vi "Detect AprilTags.vi"() -> ()   [LabVIEW 2020, in "examples.lvlib"]
doc: "Demonstrate the AprilTag Detector and the utilities for getting AprilTag Family Image Data."
uses:
  examples.lvlib
  feature_detection/Apriltag Detector/AprilTag Detector.lvclass/AprilTag Detector.ctl
  feature_detection/Apriltag Detector/AprilTag Detector.lvclass
  image/image.lvlib
  image/ARGB Colour.ctl
  feature_detection/feature_detection.lvlib
  image/Draw Poly Lines (ARGB).vi
  image/Draw Image to Picture (ARGB).vi
  image/New Image (ARGB Preallocated).vi
  feature_detection/Apriltag Detector/Create (Tag36h11).vi
  image/Horizontal Concat Image Data (ARGB).vi
  feature_detection/AprilTag ID List (Tag36h11).vi
  feature_detection/Generate Apriltag Image Data (Tag36h11).vi
  image/New Image (Greyscale Array).vi
  common/Image Point (Float).ctl
  common/common.lvlib
  common/Quad Corners.ctl
  feature_detection/Apriltag Detector/Detection.ctl
  feature_detection/Apriltag Detector/Time Profiler Entry.ctl
panel:
  out "Time Profile Entries":T1[](array[typedef])
  out "Picture":picture
  out "Detections":T2[](array[typedef])
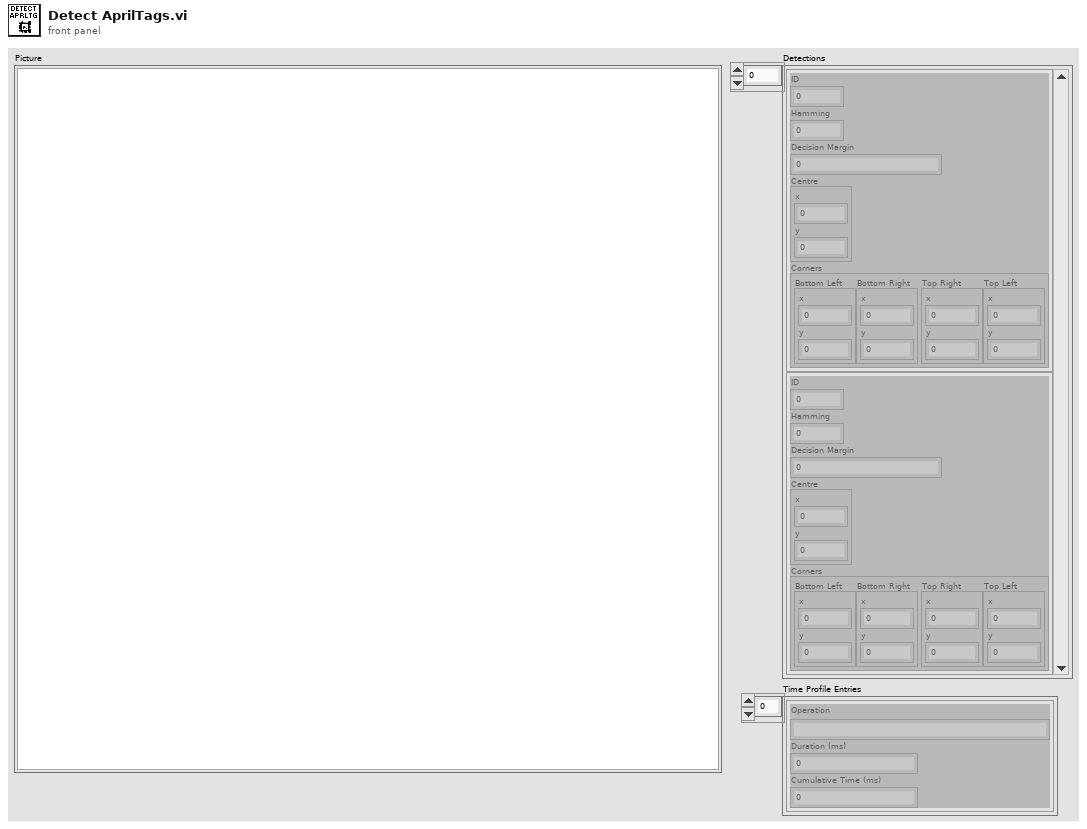
[diagram p1: front panel]
types:
  T1 = typedef "feature_detection.lvlib/AprilTag Detector.lvclass/Time Profiler Entry.ctl" = cluster{"Operation":string, "Duration (ms)":dbl, "Cumulative Time (ms)":dbl}
  T2 = typedef "feature_detection.lvlib/AprilTag Detector.lvclass/Detection.ctl" = cluster{"ID":i32, "Hamming":i32, "Decision Margin":sgl, "Centre":T3, "Corners":T4}
  T3 = typedef "common.lvlib/Image Point (Float).ctl" = cluster{"x":dbl, "y":dbl}
  T4 = typedef "common.lvlib/Quad Corners.ctl" = cluster{"Bottom Left":T3, "Bottom Right":T3, "Top Right":T3, "Top Left":T3}
  T5 = typedef "image.lvlib/ARGB Colour.ctl" = cluster{"Alpha":u8, "RGB":u32}
  T6 = typedef "image.lvlib/Greyscale Image.ctl" = refnum<data-value>
  T7 = typedef "image.lvlib/ARGB Image.ctl" = refnum<data-value>
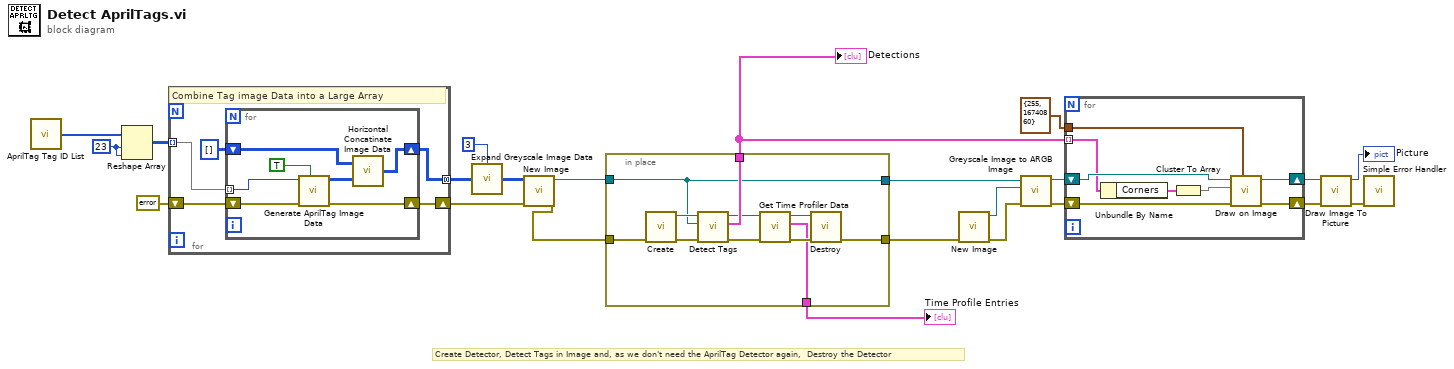
[diagram p0: block diagram]
diagram:
  w8 = 23 ("dimension size")
  # "Create Detector, Detect Tags in Image and, as we don't need the AprilTag Detector again,  Destroy the Detector"
  n1 = call-poly "AprilTag Tag ID List.vi"() -> ("Tag IDs"=w10:i32[])
  n2 = Reshape Array(w10, w8, w8) -> (w9:i32[][])
  n3 = for {
    tunnel: w9 -> [w28] mode=indexing
    tunnel: [w24] -> w6 mode=concatenating
    shift-right: [w26] -> w7
    shift-left: errorcluster {"status"=FALSE, "code"=0, "source"=""} ("error out") -> [w27]
    # "Combine Tag image Data into a Large Array"
    n4 = for {
      tunnel: w28 -> [w35] mode=indexing
      shift-right: [w33] -> w26
      shift-left: w27 -> [w34]
      shift-right: [w29] -> w24
      shift-left: u8[][] [] ("A") -> [w30]
      n5 = call-poly "Generate AprilTag Image Data.vi"("Add Border (Default: False)"=TRUE, "error in (no error)"=w34, "ID"=w35) -> ("error out"=w33:errorcluster, "Tag Image Data"=w31:u8[][])  [unwired: 7 in]
      n6 = call-poly "Horizontal Concatinate Image Data.vi"("B"=w31, "A"=w30) -> ("A Horizontal Concatinated with B"=w29:u8[][])
    }
  }
  n7 = call "Expand Greyscale Image Data.vi"("Greyscale Data"=w6, "Factor"=u16 3) -> ("Expanded Greyscale Data"=w5:u8[][])
  n8 = call-poly "New Image.vi"("error in (no error)"=w7, "U8 Greyscale Data"=w5) -> ("error out"=w23:errorcluster, "Greyscale Image"=w22:T6)  [unwired: 8 in]
  n9 = in-place {
    in-place-border: w23 -> [w45]
    in-place-border: w22 -> [w41]
    in-place-border: [w44] -> w21
    in-place-border: [w43] -> w16
    in-place-border: [w41] -> w2
    in-place-border: [w36] -> w1
    n10 = call-poly "Create.vi"("error in (no error)"=w45) -> ("error out"=w42:errorcluster, "Apriltag Detector"=w46:refnum<class "AprilTag Detector.lvclass">)  [unwired: 9 in]
    n11 = call "Detect Tags.vi"("error in (no error)"=w42, "Greyscale Image in"=w41, "Apriltag Detector in"=w46) -> ("error out"=w39:errorcluster, "Detections"=w43:T2[], "Apriltag Detector"=w40:refnum<class "AprilTag Detector.lvclass">)  [unwired: 5 in, 1 out]
    n12 = call "Get Time Profiler Data.vi"("error in (no error)"=w39, "Apriltag Detector in"=w40) -> ("error out"=w37:errorcluster, "Time Profile Entries"=w36:T1[], "Apriltag Detector"=w38:refnum<class "AprilTag Detector.lvclass">)  [unwired: 7 in]
    n13 = call "Destroy.vi"("error in (no error)"=w37, "Apriltag Detector in"=w38) -> ("error out"=w44:errorcluster)  [unwired: 9 in]
  }
  "Detections" <- w16
  "Time Profile Entries" <- w1
  n14 = call-poly "New Image.vi"("error in (no error)"=w21) -> ("error out"=w18:errorcluster, "ARGB Image"=w20:T7)  [unwired: 9 in]
  n15 = call "Greyscale Image to ARGB Image.vi"("error in (no error)"=w18, "ARGB Image Destination in"=w20, "Greyscale Image Source in"=w2) -> ("error out"=w17:errorcluster, "ARGB Image Destination"=w19:T7)  [unwired: 7 in]
  n16 = for {
    shift-right: [w52] -> w14
    shift-left: w19 -> [w54]
    tunnel: w16 -> [w51] mode=indexing
    shift-right: [w49] -> w15
    shift-left: w17 -> [w53]
    tunnel: T5 {"Alpha"=255, "RGB"=16740860} ("ARGB Colour") -> [w47]
    n17 = Unbundle By Name(w51) -> ("Corners"=w50:T4)
    n18 = Cluster To Array(cluster=w50) -> (array=w48:T3[])
    n19 = call-poly "Draw on Image.vi"("ARGB Colour"=w47, "error in (no error)"=w53, "Points"=w48, "ARGB Image in"=w54) -> ("error out"=w49:errorcluster, "ARGB Image"=w52:T7)  [unwired: 6 in]
  }
  n20 = call-poly "Draw Image To Picture.vi"("error in (no error)"=w15, "ARGB Image Source in"=w14) -> ("error out"=w13:errorcluster, "Picture"=→"Picture":picture)  [unwired: 8 in]
  n21 = call <vilib>:"Simple Error Handler.vi"("error in (no error)"=w13) -> ()  [unwired: 4 in, 5 out]
